vi "Construct.vi"(8 "error in (no error)":errorcluster) -> (0 "error out":errorcluster, 3 "Exit out":refnum<class "Exit.lvclass">)   [LabVIEW 2020, in "UpstreamMsg.lvlib" / "Exit.lvclass"]
uses:
  Exit.lvclass
  Exit.lvclass/Exit.ctl
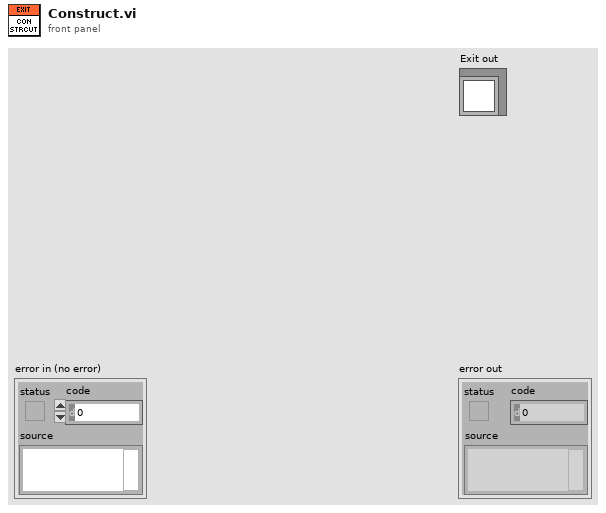
[diagram p1: front panel]
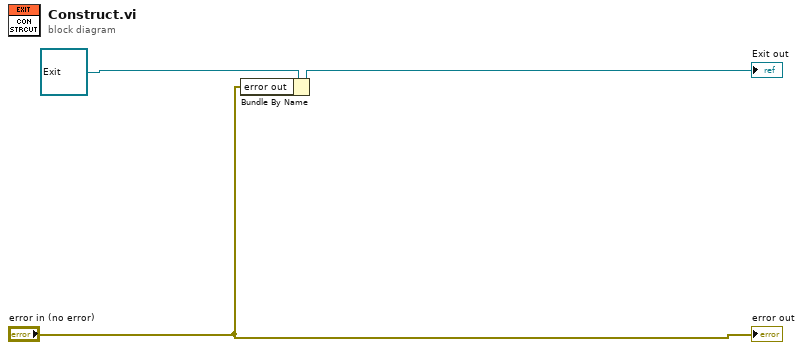
[diagram p0: block diagram]
diagram:
  n1 = Bundle By Name(cluster=refnum<class "Exit.lvclass"> refnum ("Exit in"), "error out"="error in (no error)") -> (→"Exit out":refnum<class "Exit.lvclass">)
  "error out" <- "error in (no error)"
